vi "AWS Keys Updater(TESTER).vi"() -> ()   [LabVIEW 2019]
doc: "Updates the AWS Access and Secret keys if a properly formatted file is received in the ~/AWS/incoming folder. \n\nThis is to do on-the-fly changes to the AWS credentials (without stopping/restarting MODAQ) and is not a subsitution to valid keys being set in the configurator."
uses:
  Globals and Definitions/System Message.ctl
  <vilib>/National Instruments/LabVIEW Interface for Amazon S3/LV Interface for Amazon S3.lvlib
panel:
  out "string":string
  out "All Files in Dir":path[](array[path])
  in  "?":bool
  in  "?":bool
  out "error out 2":errorcluster
  out "error out":errorcluster
  out "Cluster":T1={"Time Stamp"=timestamp(0 s since 1904-01-01), "Message Tag"="", "Message Body"="", "Snooze Time (s)"=0.0, "Snooze Alert?"=TRUE, "Log Event?"=TRUE, "Send Email"=0}
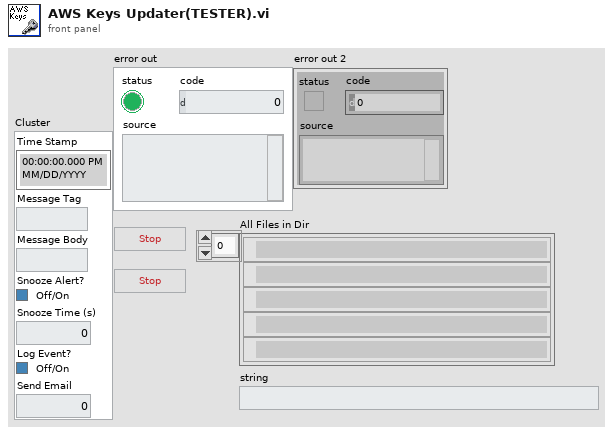
[diagram p1: front panel]
types:
  T1 = typedef "System Message.ctl" = cluster{"Time Stamp":timestamp, "Message Tag":string, "Message Body":string, "Snooze Time (s)":dbl, "Snooze Alert?":bool, "Log Event?":bool, "Send Email":i32}
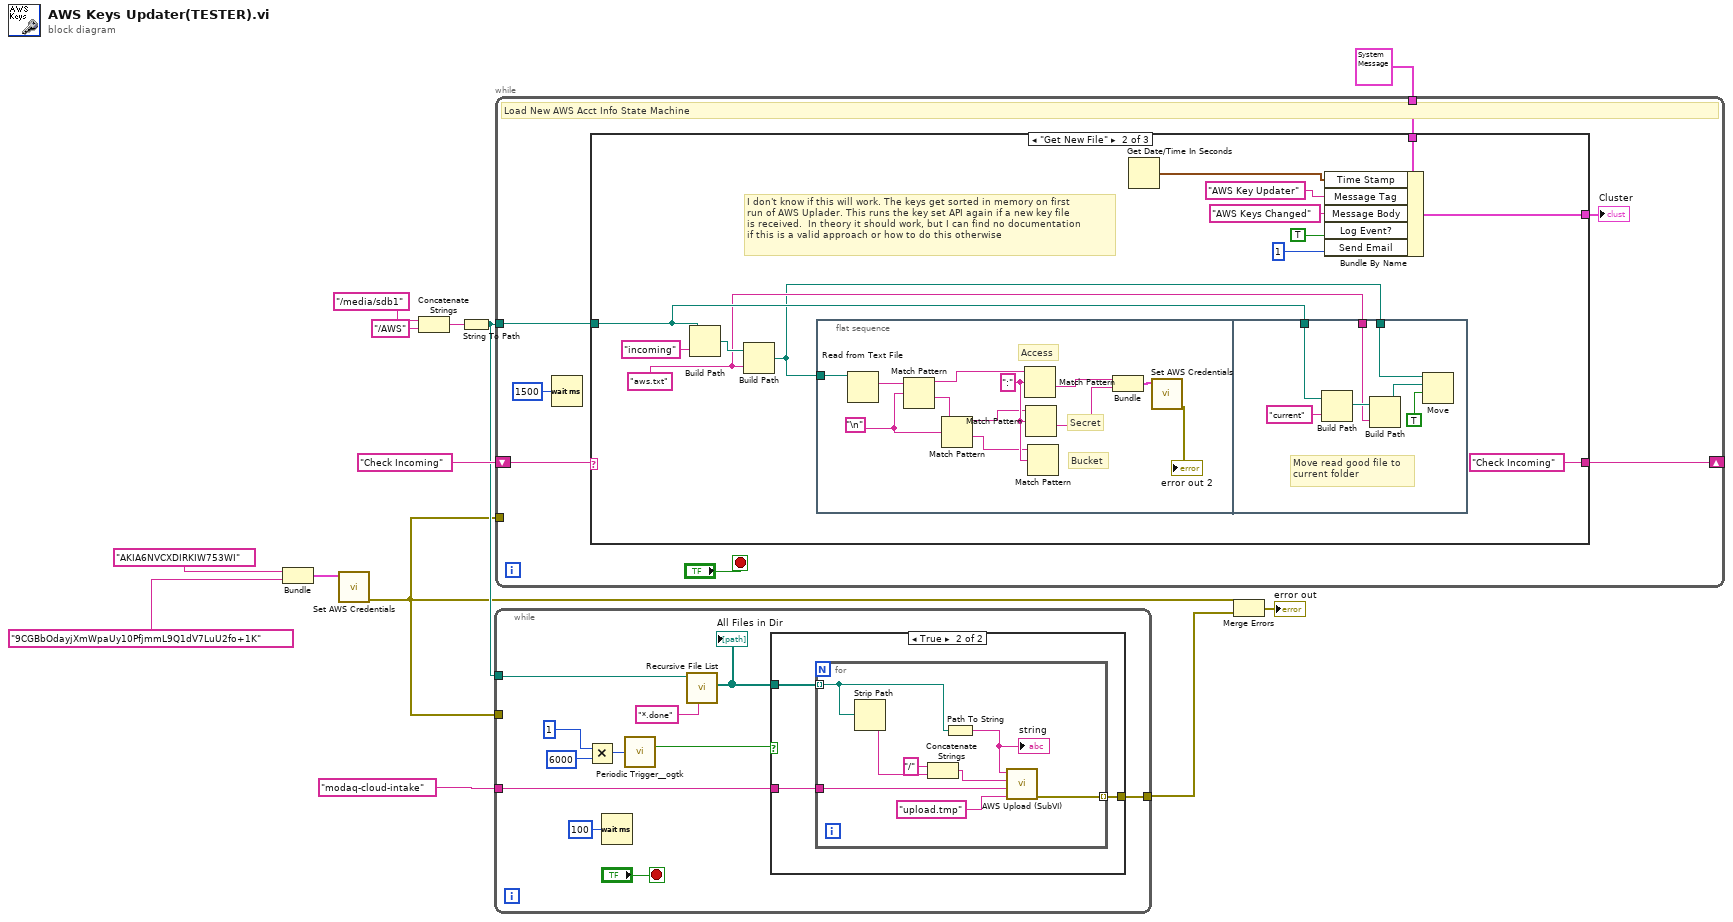
[diagram p0: block diagram]
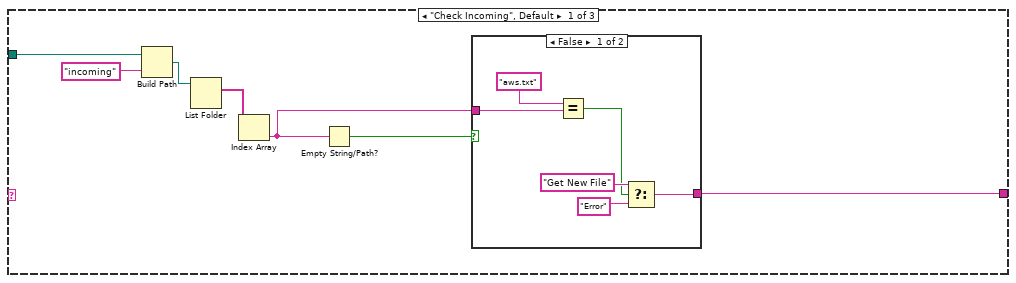
[diagram p3: hidden frame]
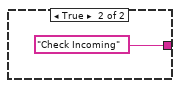
[diagram p4: hidden frame]
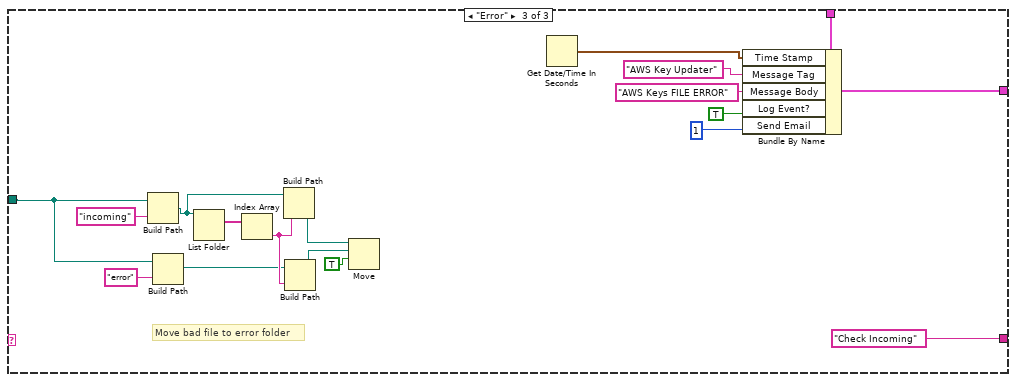
[diagram p5: hidden frame]
diagram:
  n1 = Bundle("AKIA6NVCXDIRKIW753WI", "9CGBbOdayjXmWpaUy10PfjmmL9Q1dV7LuU2fo+1K") -> (w8:cluster{string, string})  [unwired: 1 in]
  n2 = call <vilib>:"Set AWS Credentials.vi"("AWS Credentials in"=w8) -> ("error out"=w7:errorcluster)  [unwired: 10 in]
  n3 = Concatenate Strings("/media/sdb1", "/AWS" ("string")) -> (w13:string)
  n4 = String To Path(string=w13) -> (path=w9:path)
  n5 = while {
    tunnel: "modaq-cloud-intake" -> [w22]
    tunnel: [w17] -> w6
    tunnel: w9 -> [w15]
    tunnel: w7 -> [_]
    stop <- "?" stop-if-true
    n6 = Multiply(x=1, y=6000) -> (x*y=w20:i32)
    n7 = Wait (ms)(milliseconds to wait=u32 100) -> ()  [unwired: 1 out]
    n8 = call <userlib>:"Periodic Trigger__ogtk.vi"("time (ms)"=w20) -> ("Triggered"=w18:bool)  [unwired: 12 in, 2 out]
    n9 = call <vilib>:"Recursive File List.vi"("pattern"="*.done", "Folder Path"=w15) -> ("All Files in Dir"=w21:path[])  [unwired: 5 in, 4 out]
    "All Files in Dir" <- w21
    n10 = case shown="True" w18 {
      tunnel: w22 -> [_ w27]
      tunnel: [_ w26] -> w17
      tunnel: w21 -> [_ w25]
      frame False {
      }
      frame True {
        n11 = for {
          tunnel: w27 -> [w33]
          tunnel: [w30] -> w26 mode=indexing
          tunnel: w25 -> [w29] mode=indexing
          n12 = Strip Path(path=w29) -> (name=w28:string)  [unwired: 1 out]
          n13 = Concatenate Strings("/" ("string"), w28) -> (w31:string)
          n14 = Path To String(path=w29) -> (string=w34:string)
          "string" <- w34
          n15 = call "AWS Upload (SubVI).vi"("Temp Filename"="upload.tmp", "AWS Bucket"=w33, "Object path"=w31, "Local File Path"=w34) -> ("error out"=w30:errorcluster)  [unwired: 6 in, 1 out]
        }
      }
    }
  }
  n16 = while {
    shift-right: [w41] -> _
    shift-left: "Check Incoming" -> [w39]
    tunnel: w9 -> [w40]
    tunnel: T1 {"Time Stamp"=timestamp(0 s since 1904-01-01), "Message Tag"="", "Message Body"="", "Snooze Time (s)"=0.0, "Snooze Alert?"=TRUE, "Log Event?"=TRUE, "Send Email"=0} -> [w38]
    tunnel: w7 -> [_]
    stop <- "?" stop-if-true
    # "Load New AWS Acct Info State Machine"
    n17 = Wait (ms)(milliseconds to wait=u32 1500) -> ()  [unwired: 1 out]
    n18 = case shown="\"Get New File\"" w39 {
      tunnel: [w43 "Check Incoming" "Check Incoming"] -> w41
      tunnel: w40 -> [w44 w67 w100]
      tunnel: w38 -> [_ w58 w90]
      tunnel: [_ w57 w89] -> w37
      frame "Check Incoming", Default {
        n19 = Build Path(base path=w44, name or relative path="incoming") -> (appended path=w47:path)
        n20 = List Folder(path=w47) -> (filenames=w49:string[])  [unwired: 3 in, 3 out]
        n21 = Index Array(array=w49) -> (element=w45:string)  [unwired: 1 in]
        n22 = Empty String/Path?(string/path=w45) -> (empty?=w46:bool)
        n23 = case shown="False" w46 {
          tunnel: [w50 "Check Incoming"] -> w43
          tunnel: w45 -> [w54 _]
          frame False {
            n24 = Equal?(x="aws.txt", y=w54) -> (x = y?=w51:bool)
            n25 = Select(t="Get New File", s=w51, f="Error") -> (s? t:f=w50:string)
          }
          frame True {
          }
        }
      }
      frame "Get New File" {
        w66 = "aws.txt"
        # "I don't know if this will work. The keys get sorted in memory on first\nrun of AWS Uplader. This runs the key set API again if a new key file\nis received.  In theory it should work, but I can find no documentation\nif this is a valid approach or how to do this otherwise"
        n26 = Build Path(base path=w67, name or relative path="incoming") -> (appended path=w68:path)
        n27 = Build Path(base path=w68, name or relative path=w66) -> (appended path=w64:path)
        n28 = flat-sequence {
          tunnel: w64 -> [w74]
          tunnel: w67 -> [w85]
          tunnel: w66 -> [w84]
          tunnel: w64 -> [w83]
          frame #0 {
            w77 = ":" ("regular expression")
            w79 = "\n"
            # "Bucket"
            # "Secret"
            # "Access"
            n29 = Read from Text File(file (use dialog)=w74) -> (text=w81:string)  [unwired: 3 in, 3 out]
            n30 = Match Pattern(string=w81, regular expression=w79) -> (before substring=w78:string, after substring=w80:string)  [unwired: 1 in, 2 out]
            n31 = Match Pattern(string=w80, regular expression=w79) -> (before substring=w76:string, after substring=w75:string)  [unwired: 1 in, 2 out]
            n32 = Match Pattern(string=w78, regular expression=w77) -> (after substring=w72:string)  [unwired: 1 in, 3 out]
            n33 = Match Pattern(string=w76, regular expression=w77) -> (after substring=w71:string)  [unwired: 1 in, 3 out]
            n34 = Match Pattern(string=w75, regular expression=w77) -> ()  [unwired: 1 in, 4 out]
            n35 = Bundle(w72, w71) -> (w73:cluster{string, string})  [unwired: 1 in]
            n36 = call <vilib>:"Set AWS Credentials.vi"("AWS Credentials in"=w73) -> ("error out"=→"error out 2":errorcluster)  [unwired: 10 in]
          }
          frame #1 {
            # "Move read good file to\ncurrent folder"
            n37 = Build Path(base path=w85, name or relative path="current") -> (appended path=w87:path)
            n38 = Build Path(base path=w87, name or relative path=w84) -> (appended path=w88:path)
            n39 = Move(source path=w83, 9:TRUE ("overwrite (F)"), 10:w88) -> ()  [unwired: 2 in, 3 out]
          }
        }
        n40 = Get Date/Time In Seconds() -> (seconds since 1Jan1904=w63:timestamp)
        n41 = Bundle By Name(cluster=w58, "Time Stamp"=w63, "Message Tag"="AWS Key Updater", "Message Body"="AWS Keys Changed", "Log Event?"=TRUE, "Send Email"=1) -> (w57:T1)
      }
      frame "Error" {
        # "Move bad file to error folder"
        n42 = Build Path(base path=w100, name or relative path="incoming") -> (appended path=w103:path)
        n43 = Build Path(base path=w100, name or relative path="error") -> (appended path=w98:path)
        n44 = List Folder(path=w103) -> (filenames=w104:string[])  [unwired: 3 in, 3 out]
        n45 = Index Array(array=w104) -> (element=w99:string)  [unwired: 1 in]
        n46 = Build Path(base path=w103, name or relative path=w99) -> (appended path=w102:path)
        n47 = Build Path(base path=w98, name or relative path=w99) -> (appended path=w97:path)
        n48 = Move(source path=w102, 9:TRUE ("overwrite (F)"), 10:w97) -> ()  [unwired: 2 in, 3 out]
        n49 = Get Date/Time In Seconds() -> (seconds since 1Jan1904=w95:timestamp)
        n50 = Bundle By Name(cluster=w90, "Time Stamp"=w95, "Message Tag"="AWS Key Updater", "Message Body"="AWS Keys FILE ERROR", "Log Event?"=TRUE, "Send Email"=1) -> (w89:T1)
      }
    }
    "Cluster" <- w37
  }
  n51 = Merge Errors(w7, w6) -> (→"error out":errorcluster)
